vi "Configure Voltage Limit.vi"(8 "error in (no error)":errorcluster, 9 "Max Voltage Limit (31.000 V)":dbl=31.0 min=0.0 max=61.0 step=0.001 format="%.3f", 10 "Channel (1:1)":u16(ring)=1 items=["1"=1, "2"=2, "3"=3], 11 "VISA resource name":refnum<visa-resource-name>) -> (0 "error out":errorcluster, 3 "VISA resource name out":refnum<visa-resource-name>)   [LabVIEW 2017, in "BK Precision 913XX.lvlib"]
doc: "Configures the maximum output voltage limit of the selected channel."
uses:
  <instrlib>/BK Precision 913XX/BK Precision 913XX.lvlib
panel:
  # "V"
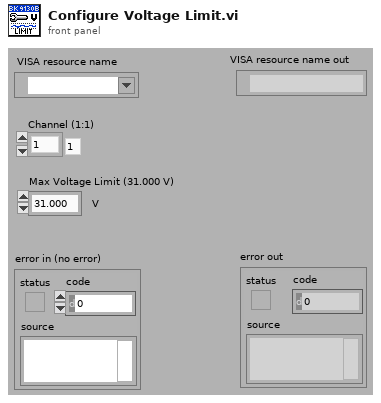
[diagram p1: front panel]
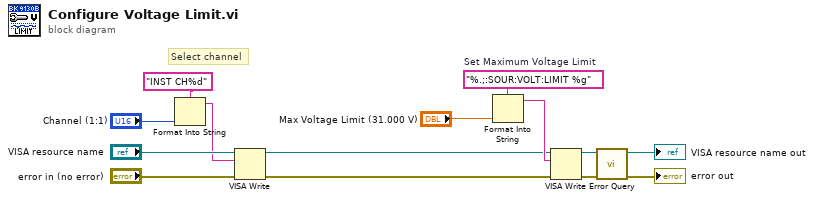
[diagram p0: block diagram]
diagram:
  w10 = "%.;:SOUR:VOLT:LIMIT %g"  # Set Maximum Voltage Limit
  # "Select channel"
  n1 = Format Into String(format string="INST CH%d", "Channel (1:1)") -> (resulting string=w2:string)  [unwired: 2 in, 1 out]
  n2 = VISA Write(VISA resource name="VISA resource name", write buffer=w2, error in (no error)="error in (no error)") -> (VISA resource name out=w4:refnum<visa-resource-name>, error out=w5:errorcluster)  [unwired: 1 out]
  n3 = Format Into String(format string=w10, "Max Voltage Limit (31.000 V)") -> (resulting string=w8:string)  [unwired: 2 in, 1 out]
  n4 = VISA Write(VISA resource name=w4, write buffer=w8, error in (no error)=w5) -> (VISA resource name out=w11:refnum<visa-resource-name>, error out=w12:errorcluster)  [unwired: 1 out]
  n5 = call <instrlib>:"Error Query.vi"("error in (no error)"=w12, "VISA resource name"=w11) -> ("error out"=→"error out":errorcluster, "VISA resource name out"=→"VISA resource name out":refnum<visa-resource-name>)  [unwired: 6 in, 2 out]
